vi "Draw.vi"(11 "Data In":T1) -> ()   [LabVIEW 2020]
uses:
  Data.ctl
panel:
  out "Grid":string[][](array[string])
  out "Score":i64
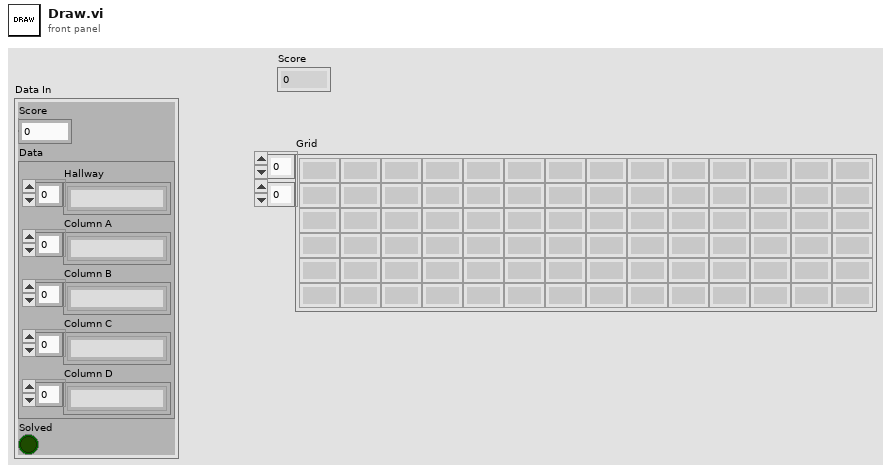
[diagram p1: front panel]
types:
  T1 = typedef "Data.ctl" = cluster{"Score":i64, "Data":cluster{"Hallway":string[], "Column A":string[], "Column B":string[], "Column C":string[], "Column D":string[]}, "Solved":bool}
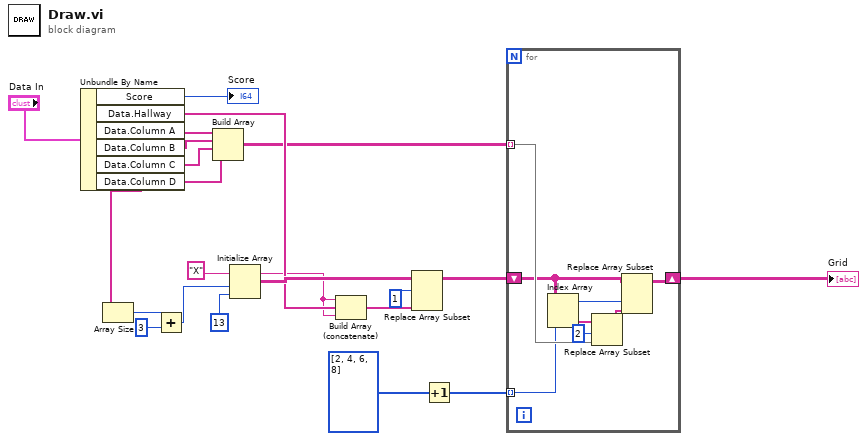
[diagram p0: block diagram]
diagram:
  w13 = "X"
  n1 = Unbundle By Name("Data In") -> ("Score"=→"Score":i64, "Data.Hallway"=w15:string[], "Data.Column A"=w7:string[], "Data.Column B"=w8:string[], "Data.Column C"=w9:string[], "Data.Column D"=w10:string[])
  n2 = Array Size(array=w10) -> (size(s)=w18:i32)
  n3 = Add(x=w18, y=3) -> (x+y=w4:i32)
  n4 = Build Array(w7, w8, w9, w10) -> (w6:string[][])
  n5 = Initialize Array(w13, w4, 13 ("dimension size")) -> (w16:string[][])
  n6 = Build Array (concatenate)(w13, w15, w13) -> (w14:string[])
  n7 = Replace Array Subset(array=w16, new element=w14, index (row)=1) -> (w12:string[][])  [unwired: 1 in]
  n8 = Increment(x=i32[] [2, 4, 6, 8]) -> (x+1=w1:i32[])
  n9 = for {
    shift-right: [w21] -> w11
    shift-left: w12 -> [w23]
    tunnel: w6 -> [w26] mode=indexing
    tunnel: w1 -> [w22] mode=indexing
    n10 = Index Array(array=w23, index (col)=w22) -> (element=w27:string[])  [unwired: 1 in]
    n11 = Replace Array Subset(array=w27, new element=w26, index=2) -> (w24:string[])
    n12 = Replace Array Subset(array=w23, new element=w24, index (col)=w22) -> (w21:string[][])  [unwired: 1 in]
  }
  "Grid" <- w11
